vi "MB_init_all.vi"() -> ()   [LabVIEW 2011]
panel:
  out "Conn. Axes out":string[](array[string])
  out "C-726.1CD":string[](array[string])
  out "C-726.1CD":dbl[](array[numeric]) format="%.6f"
  out "C843\nPosition":dbl[](array[numeric]) format="%.6f"
  out "C843\nConn. \nAxis":string[](array[string])
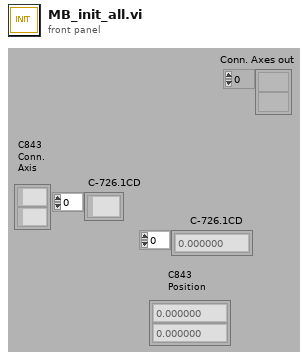
[diagram p1: front panel]
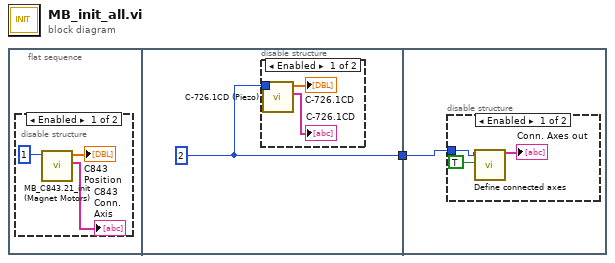
[diagram p0: block diagram]
diagram:
  n1 = flat-sequence {
    tunnel: [w5] -> w1
    tunnel: w1 -> [w9]
    frame #0 {
      n2 = disable-structure shown="Enabled" {
        frame Enabled {
          n3 = call "MB_C843.21_init (Magnet Motors).vi"("System no."=1) -> ("C843\nConn. \nAxis"=→"C843\nConn. \nAxis":string[], "Position"=→"C843\nPosition":dbl[])  [unwired: 9 out]
        }
        frame Disabled {
        }
      }
    }
    frame #1 {
      w5 = 2 ("System no.")
      n4 = disable-structure shown="Enabled" {
        disable-tunnel: w5 -> [w6 _]
        frame Enabled {
          n5 = call "C-726.1CD (Piezo).vi"("System no."=w6) -> ("Conn. Axis"=→"C-726.1CD":string[], "C-726.1CD"=→"C-726.1CD":dbl[])  [unwired: 1 in, 8 out]
        }
        frame Disabled {
        }
      }
    }
    frame #2 {
      n6 = disable-structure shown="Enabled" {
        disable-tunnel: w9 -> [w10 _]
        frame Enabled {
          n7 = call "Define connected axes.vi"("System no."=w10, "Read from\ncontroller?"=TRUE ("Read from\ncontroller?")) -> ("Conn. Axes out"=→"Conn. Axes out":string[])  [unwired: 16 in, 1 out]
        }
        frame Disabled {
        }
      }
    }
  }
